vi "camera up and down thing.vi"(8 "error in (no error)":errorcluster, 10 "down button":bool, 11 "up button":bool) -> (0 "error out":errorcluster)   [LabVIEW 2014]
uses:
  <vilib>/Rock Robotics/WPI/Relay/WPI_RelayValue.ctl
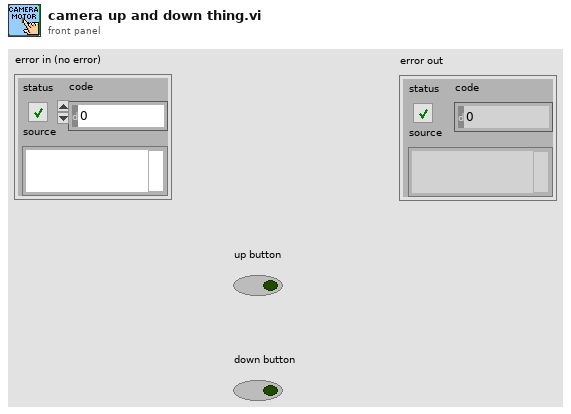
[diagram p1: front panel]
types:
  T1 = typedef "WPI_RelayValue.ctl" = enum16{"Off", "On", "Forward", "Reverse"}
  T2 = typedef "WPI_RelayDevRef.ctl" = cluster{"DevStatus":errorcluster, "Relay Channel":T3, "Controller":T4, "Relay Direction":T5}
  T3 = typedef "FPGA_DIORelayChannel.ctl" = enum8{"Relay 0", "Relay 1", "Relay 2", "Relay 3", "Invalid"}
  T4 = typedef "FPGA_TypedefDigitalModule.ctl" = enum16{"Controller 1"}
  T5 = typedef "WPI_RelayDirection.ctl" = enum16{"Both directions", "Forward only", "Reverse only"}
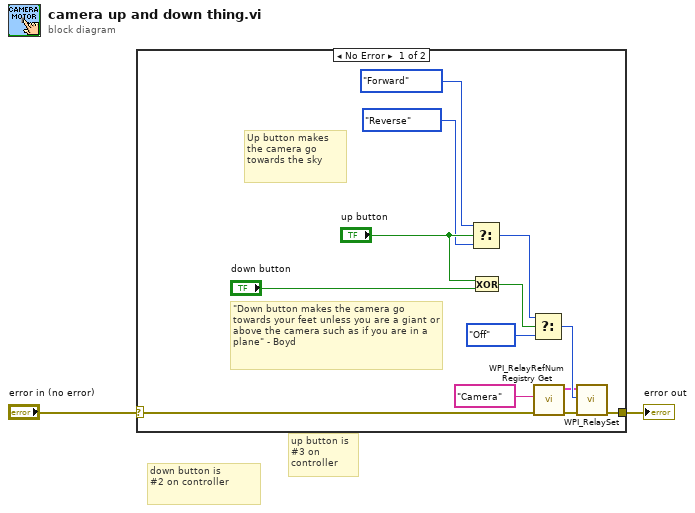
[diagram p0: block diagram]
diagram:
  # "down button is \n#2 on controller"
  # "up button is #3 on controller"
  n1 = case shown="No Error" "error in (no error)" {
    selector: "error in (no error)" -> [w5 w16]
    tunnel: [w3 w16] -> w2
    frame No Error {
      # "\"Down button makes the camera go towards your feet unless you are a giant or above the camera such as if you are in a plane\" - Boyd"
      # "Up button makes the camera go towards the sky"
      n2 = Select(t=WPI_RelayValue."Forward" ("RelayValue"), s="up button", f=WPI_RelayValue."Reverse" ("RelayValue")) -> (s? t:f=w11:T1)
      n3 = Exclusive Or(1:"down button", 2:"up button") -> (0:w13:bool)
      n4 = Select(t=w11, s=w13, f=WPI_RelayValue."Off" ("RelayValue")) -> (s? t:f=w7:T1)
      n5 = call <vilib>:"WPI_RelayRefNum Registry Get.vi"("error in (no error)"=w5, "refnum name"="Camera") -> ("error out"=w4:errorcluster, "RelayDevRef"=w6:T2)  [unwired: 8 in]
      n6 = call <vilib>:"WPI_RelaySet.vi"("error in (no error)"=w4, "RelayValue"=w7, "RelayDevRef"=w6) -> ("error out"=w3:errorcluster)  [unwired: 7 in, 1 out]
    }
    frame Error {
      # "This is what to do if there is an error.  Usually it is nothing."
    }
  }
  "error out" <- w2
